vi "Ethernet TCP Engine.vi"(8 "error in (no error)":errorcluster, 9 "Mode":u8, 10 "Engine Name":string, 11 "Varient Data":variant) -> (0 "error out":errorcluster)   [LabVIEW 2024]
doc: "All Rights Reserved © 2023 SyncSols"
uses:
  Main Engine/Controls/Main Engine Engine No.Options.ctl
  TCP Engine/Controls/TCP Engine Serial Interupt Cluster.ctl
  TCP Engine/TCP Engine.lvlib
  Main Engine/Controls/Main Engine Config Confirmation Cluster.ctl
  Controls/Ethernet Dynamic Data Cluster.ctl
  Controls/Ethernet Message Info Cluster.ctl
  Controls/Ethernet Frame Info Cluster.ctl
  Controls/Ethernet Configuration Cluster.ctl
  Controls/Ethernet Command Q Cluster.ctl
  Controls/Ethernet TCP Read Write References.ctl
  Controls/Ethernet State Machine Cases.ctl
  Controls/Ethernet Client Info Cluster.ctl
  Controls/Ethernet Server Listen Loop Cluster.ctl
  Controls/Ethernet Client Info Q Cluster.ctl
  Main Engine/Controls/Main Engine Q Option.ctl
  Main Engine/Controls/Main Engine JSON Command State.ctl
  Controls/Ethernet TCP State Machine Data Cluster.ctl
panel:
  in  "Data Cluster":T1={"Varient Data"=variant(string ""), "Stop Notification"=refnum, "Start Notification"=refnum, "Main Engine Response Q"=refnum, "TCP Engine Response Q"=refnum, "Engine Name"="", "Log File Refnum"=refnum, "Interupt Q"=refnum, "Mode"=0, "Ethernet Configuration"={"Mode"=255, "Local IP"="", "Local Port"=8, "Frame Info"=[], "Minor Frame Freq"=0}, "UDP Connection ID"=refnum, "Command Q"=refnum, "TCP Connection ID"=refnum, "Listener ID"=refnum, "Wait for Listner"=FALSE, "Remote address"=[], "Remote port"=[], "Connection ID"=[], "Client IP"="", "Client Port"=0, "Client Info Q"=refnum, "Server Listen Loop Q"=refnum}
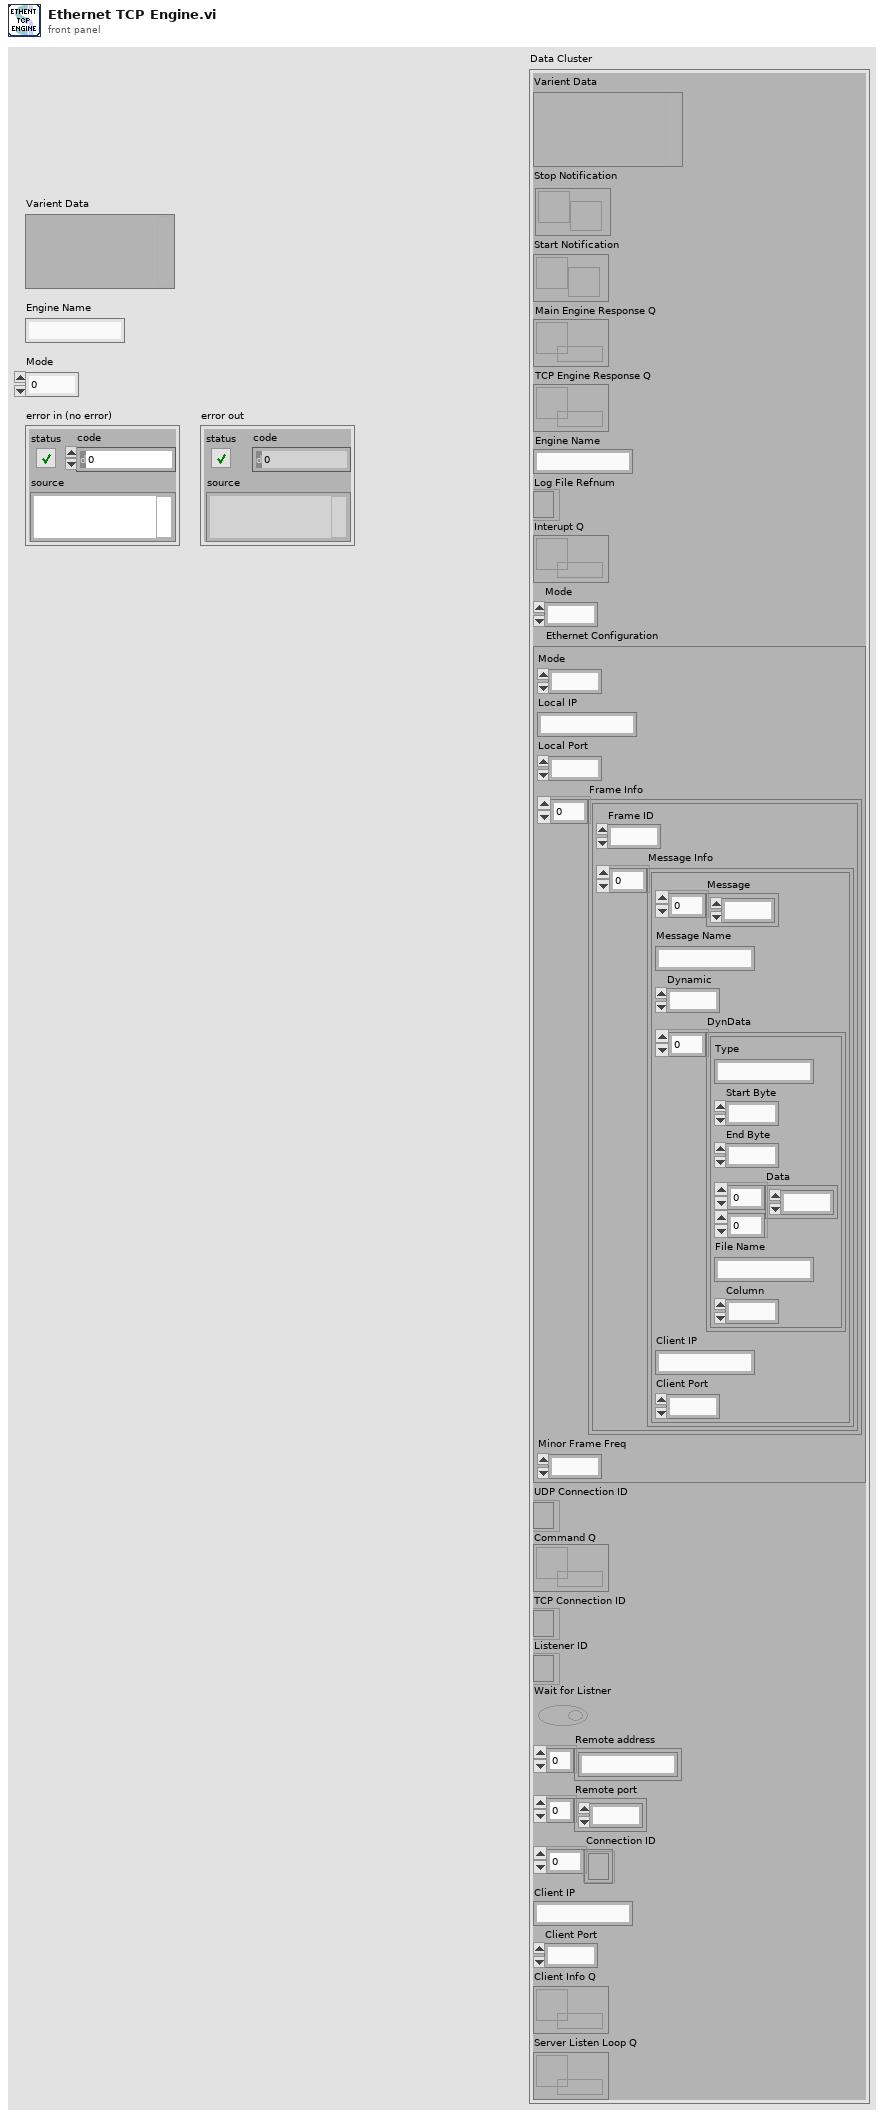
[diagram p1: front panel]
types:
  T1 = typedef "Ethernet TCP State Machine Data Cluster.ctl" = cluster{"Varient Data":variant, "Stop Notification":refnum<notifier>, "Start Notification":refnum<notifier>, "Main Engine Response Q":refnum<queue>, "TCP Engine Response Q":refnum<queue>, "Engine Name":string, "Log File Refnum":refnum<file>, "Interupt Q":refnum<queue>, "Mode":u8, "Ethernet Configuration":T2, "UDP Connection ID":refnum<k16>, "Command Q":refnum<queue>, "TCP Connection ID":refnum<k5>, "Listener ID":refnum<k5>, "Wait for Listner":bool, "Remote address":string[], "Remote port":u16[], "Connection ID":refnum<k5>[], "Client IP":string, "Client Port":u16, "Client Info Q":refnum<queue>, "Server Listen Loop Q":refnum<queue>}
  T2 = typedef "Ethernet Configuration Cluster.ctl" = cluster{"Mode":u8, "Local IP":string, "Local Port":u16, "Frame Info":T3[], "Minor Frame Freq":u8}
  T3 = typedef "Ethernet Frame Info Cluster.ctl" = cluster{"Frame ID":u16, "Message Info":T4[]}
  T4 = typedef "Ethernet Message Info Cluster.ctl" = cluster{"Message":u8[], "Message Name":string, "Dynamic":u8, "DynData":T5[], "Client IP":string, "Client Port":u16}
  T5 = typedef "Ethernet Dynamic Data Cluster.ctl" = cluster{"Type":string, "Start Byte":u8, "End Byte":u8, "Data":u32[][], "File Name":string, "Column":i32}
  T6 = typedef "Ethernet State Machine Cases.ctl" = enum16{">Poll", ".........State Machine.........", ">Init", ">Error", ">Exit", "..........Async Serial..........", ">JSON to LVData", ">Gen Dyn Data", ">Configure", ">Wait for Listener", ">Get Command", ">Write Data"}
  T7 = typedef "Ethernet Server Listen Loop Cluster.ctl" = cluster{"Local IP":string, "References":T8, "Server":bool, "Local Port":u16}
  T8 = typedef "Ethernet TCP Read Write References.ctl" = cluster{"TCP Connection ID":refnum<k5>, "TCP Engine Response Q":refnum<queue>, "Interupt Q":refnum<queue>, "Main Engine Response Q":refnum<queue>, "Stop Notification":refnum<notifier>, "Client Info Q":refnum<queue>}
  T9 = typedef "Main Engine.lvlib/Main Engine Q Option.ctl" = enum16{"Init", "Get"}
  T10 = typedef "Ethernet Client Info Q Cluster.ctl" = cluster{"TCP  ID":refnum<k5>, "Remote port":u16, "Remote IP":string}
  T11 = typedef "TCP Engine.lvlib/TCP Engine Serial Interupt Cluster.ctl" = cluster{"Stop":bool, "JSON Variant":variant}
  T12 = typedef "Ethernet Command Q Cluster.ctl" = cluster{"Ethernet Configuration":T2, "Command State":T13}
  T13 = typedef "Main Engine JSON Command State.ctl" = enum16{"Configure", "Start", "Exit"}
  T14 = typedef "Main Engine.lvlib/Main Engine Engine No.Options.ctl" = enum16{"Init", "Update", "Response", "Get"}
  T15 = typedef "Main Engine.lvlib/Main Engine Config Confirmation Cluster.ctl" = cluster{"Command":string, "Interface":string, "Status":string, "Board":string}
  T16 = typedef "Ethernet Client Info Cluster.ctl" = cluster{"Remote port":u16, "Remote IP":string, "Local port":u16, "Local address":string}
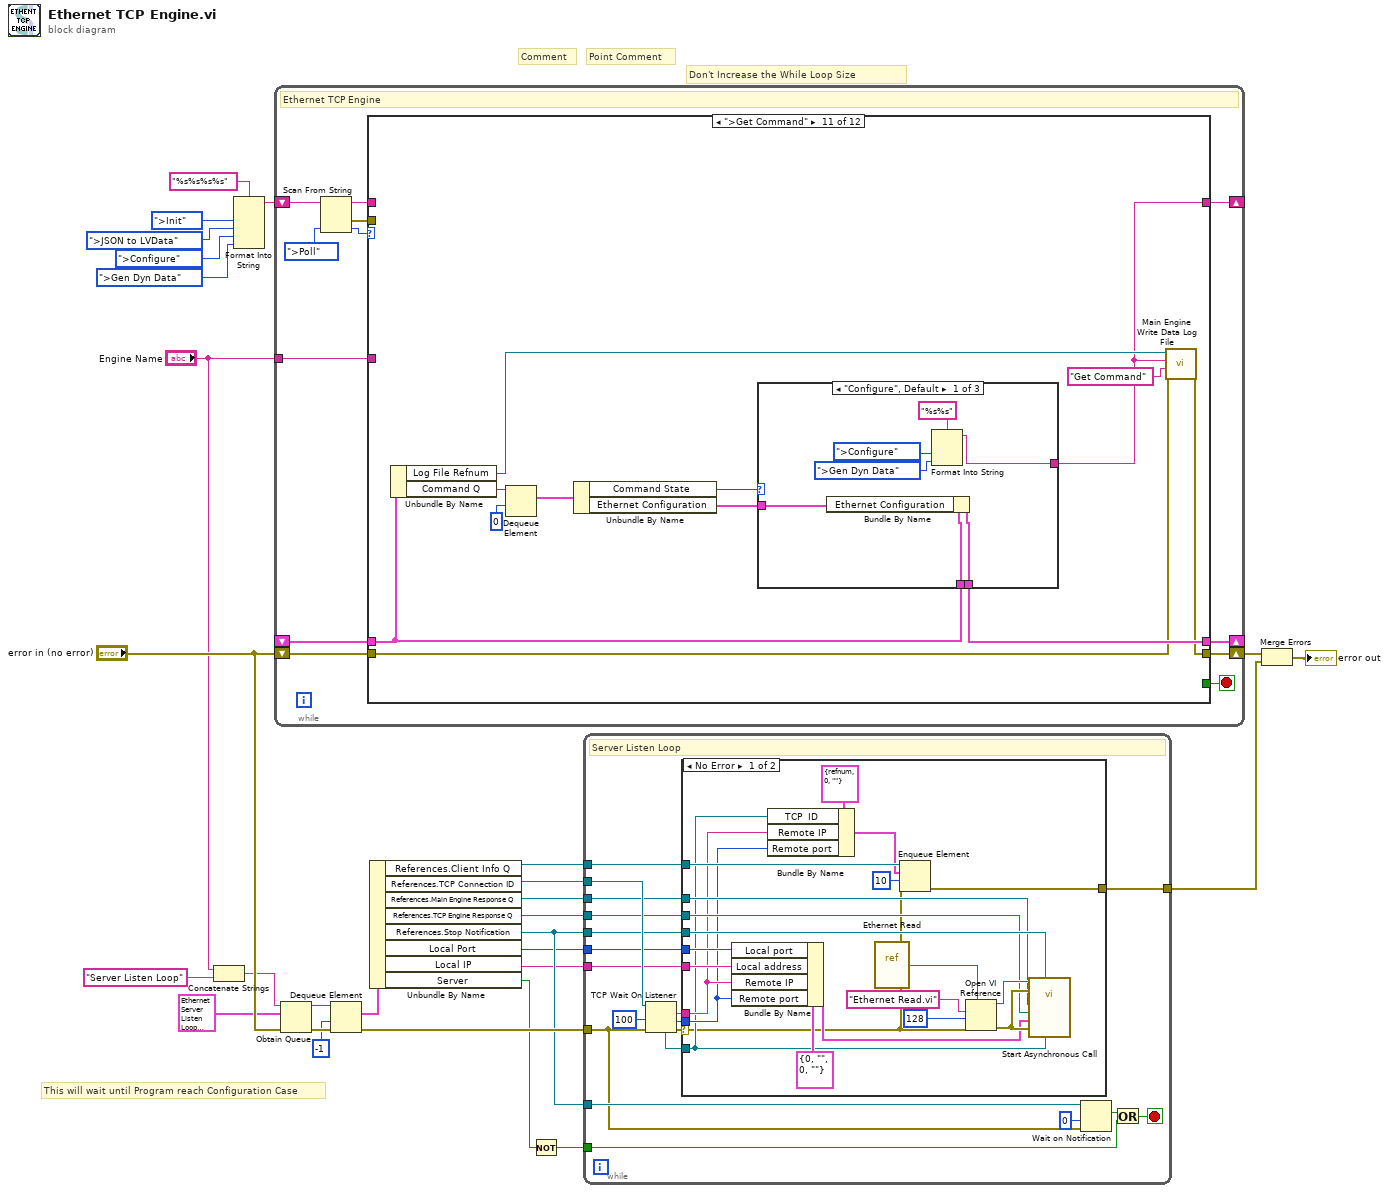
[diagram p0: block diagram]
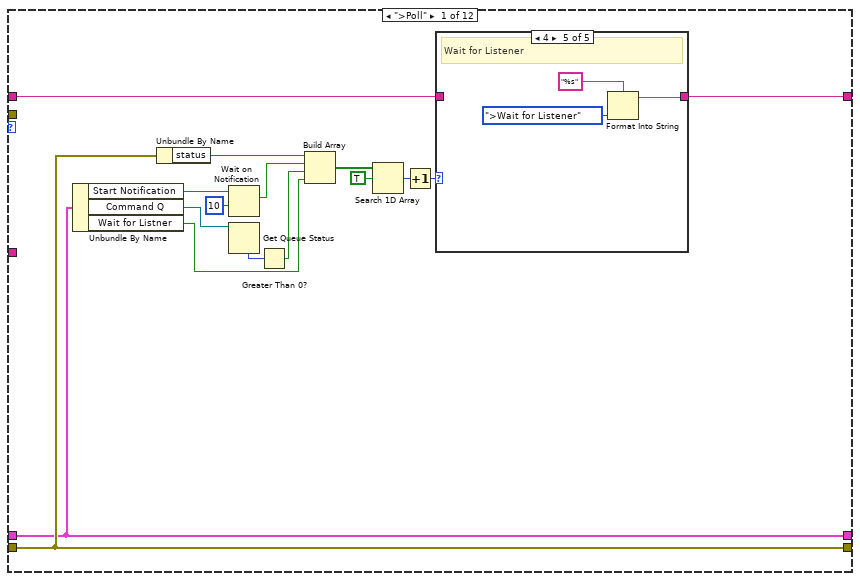
[diagram p3: hidden frame]
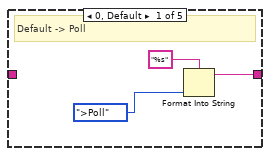
[diagram p4: hidden frame]
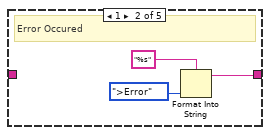
[diagram p5: hidden frame]
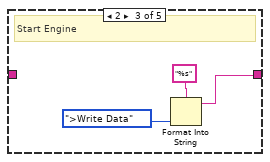
[diagram p6: hidden frame]
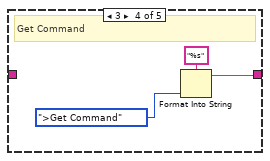
[diagram p7: hidden frame]
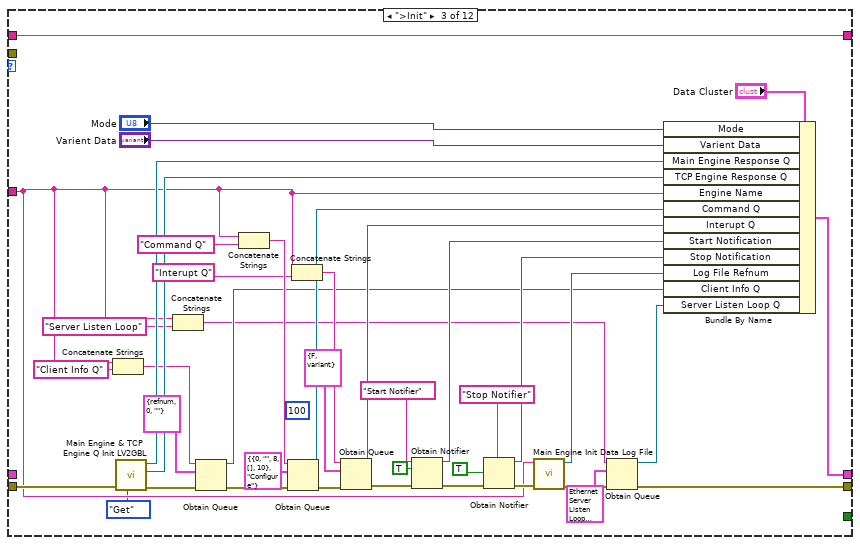
[diagram p9: hidden frame]
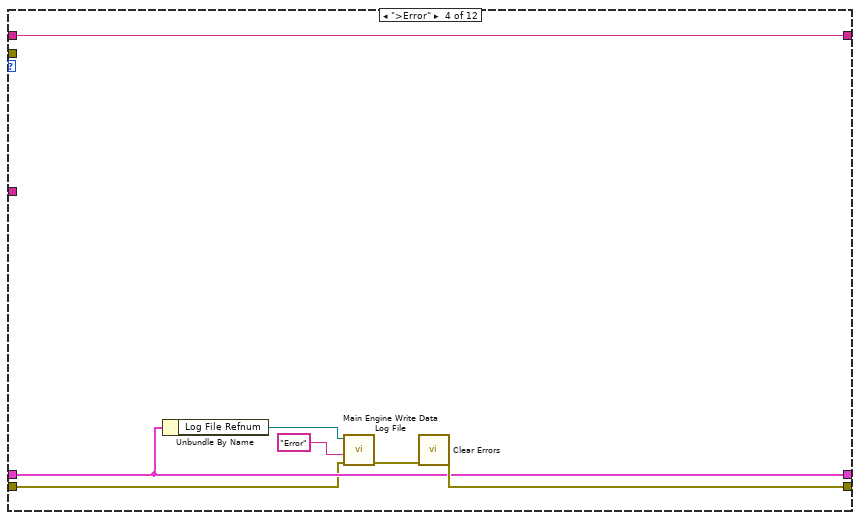
[diagram p10: hidden frame]
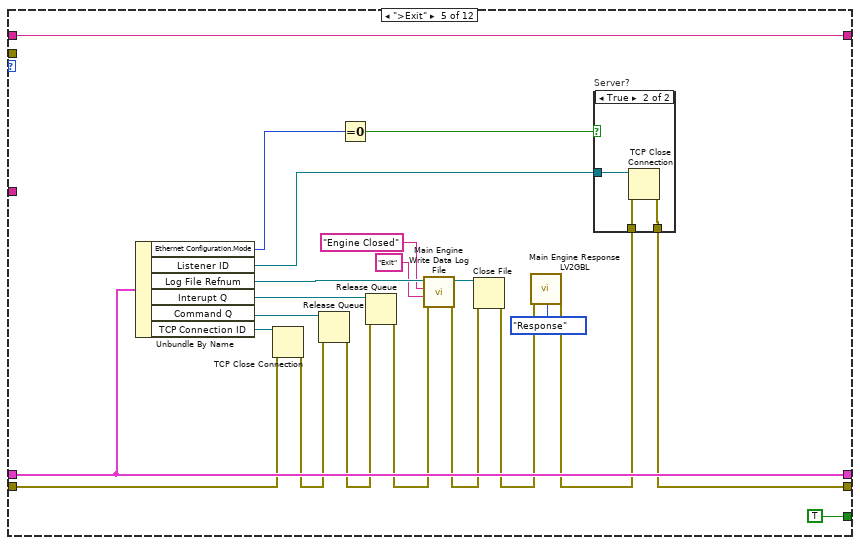
[diagram p11: hidden frame]
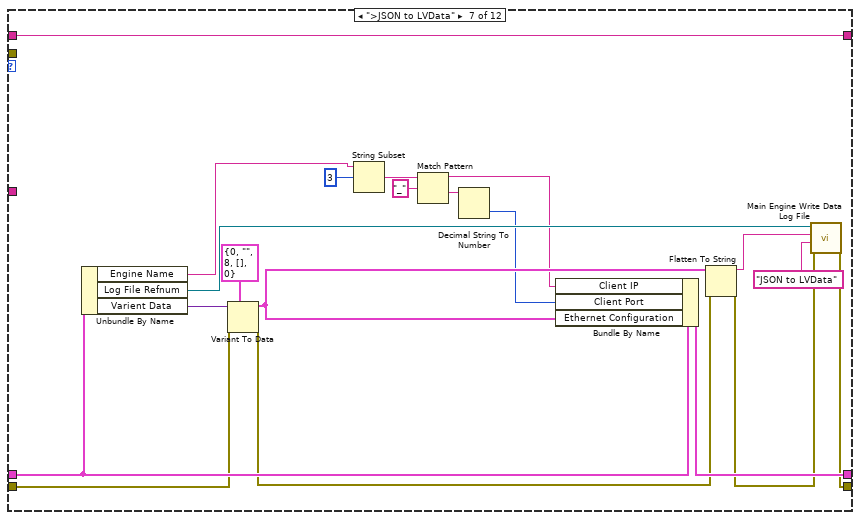
[diagram p14: hidden frame]
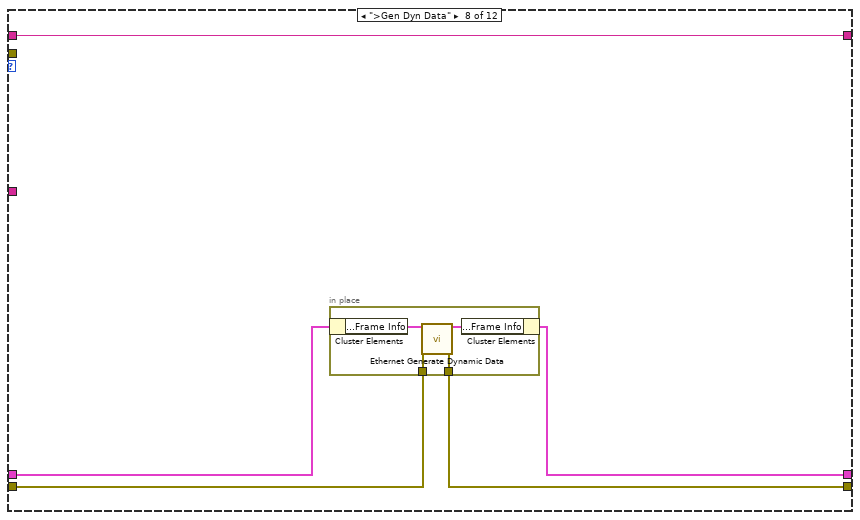
[diagram p15: hidden frame]
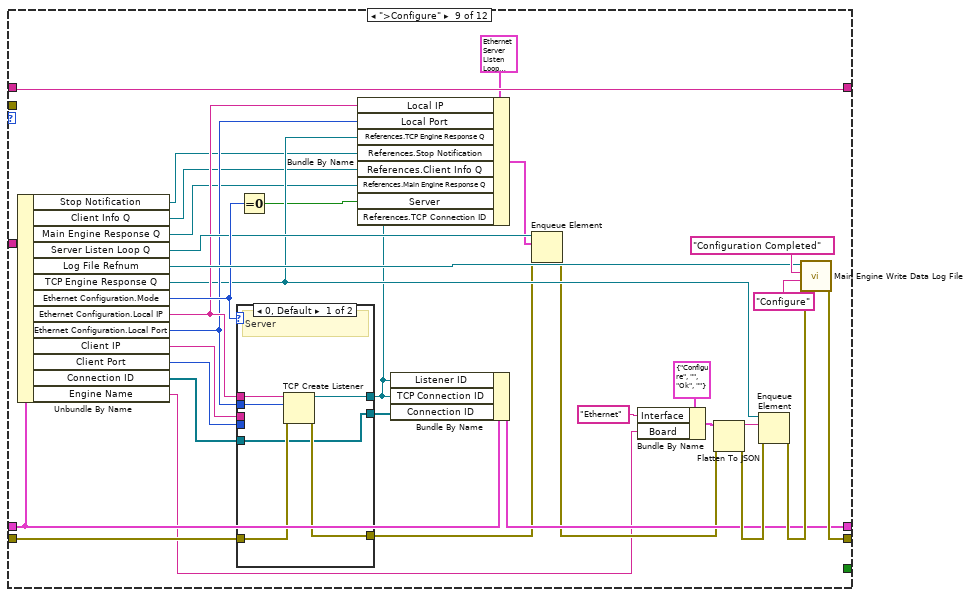
[diagram p16: hidden frame]
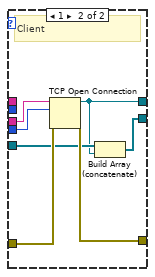
[diagram p17: hidden frame]
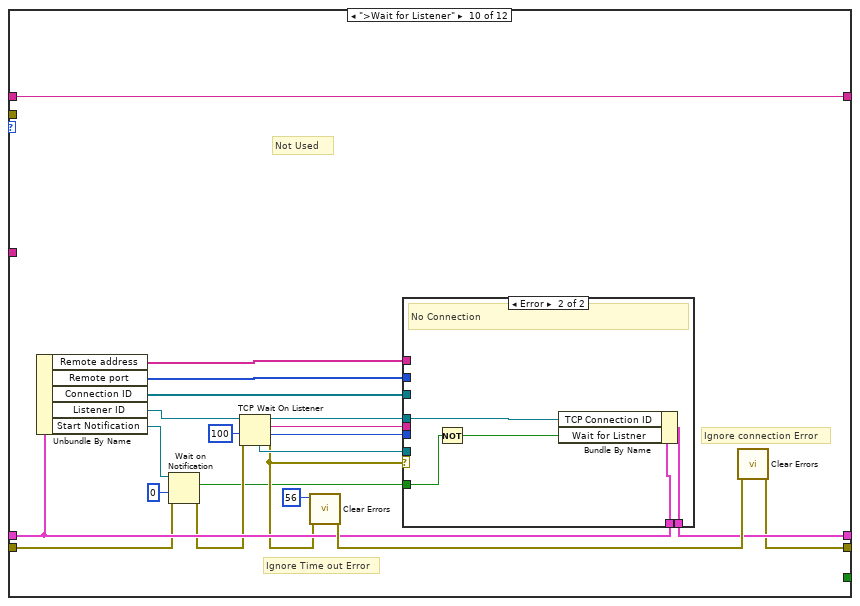
[diagram p18: hidden frame]
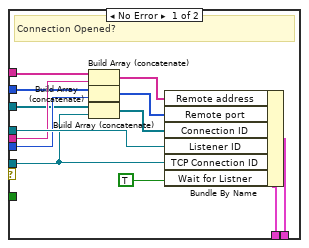
[diagram p19: hidden frame]
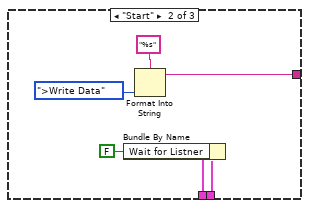
[diagram p20: hidden frame]
diagram:
  # "This will wait until Program reach Configuration Case"
  # "Don't Increase the While Loop Size"
  # "Point Comment"
  # "Comment"
  n1 = Concatenate Strings("Engine Name", "Server Listen Loop" ("string")) -> (w17:string)
  n2 = Format Into String(format string="%s%s%s%s", Ethernet_State_Machine_Cases.">Init" ("SM Cases Options"), Ethernet_State_Machine_Cases.">JSON to LVData" ("SM Cases Options"), Ethernet_State_Machine_Cases.">Configure" ("SM Cases Options"), Ethernet_State_Machine_Cases.">Gen Dyn Data" ("SM Cases Options")) -> (resulting string=w27:string)  [unwired: 2 in, 1 out]
  n3 = while {
    shift-right: [w36] -> _
    shift-left: w27 -> [w40]
    shift-right: [w34] -> w25
    shift-left: "error in (no error)" -> [w35]
    shift-right: [w32] -> _
    shift-left: _ -> [w31]
    tunnel: "Engine Name" -> [w29]
    stop <- w33 stop-if-true
    # "Ethernet TCP Engine"
    n4 = Scan From String(input string=w40, default 1=Ethernet_State_Machine_Cases.">Poll" ("SM Cases Options")) -> (remaining string=w37:string, error out=w39:errorcluster, output 1=w38:T6)  [unwired: 3 in, 1 out]
    n5 = case shown="\">Get Command\"" w38 {
      tunnel: w39 -> [_ _ _ _ _ _ _ _ _ _ _ _]
      tunnel: w37 -> [w56 w74 w115 w122 w144 w151 w171 w176 w195 w247 _ w334]
      tunnel: [w55 w74 w115 w122 w144 w151 w171 w176 w195 w247 w269 w334] -> w36
      tunnel: w35 -> [w54 w73 w93 w117 w134 w150 w161 w174 w202 w235 w266 w327]
      tunnel: [w54 w73 w77 w121 w123 w150 w166 w172 w211 w238 w267 w332] -> w34
      tunnel: [_ _ _ _ TRUE _ _ _ _ _ _ _] -> w33
      tunnel: [w48 w72 w100 w118 w142 w149 w168 w173 w201 w239 w272 w333] -> w32
      tunnel: w31 -> [w48 w72 _ w118 w142 w149 w170 w175 w213 w240 w271 w333]
      tunnel: w29 -> [_ _ w79 _ _ _ _ _ _ _ _ _]
      frame ">Poll" {
        n6 = Unbundle By Name(w48) -> ("Start Notification"=w47:refnum<notifier>, "Command Q"=w46:refnum<queue>, "Wait for Listner"=w41:bool)
        n7 = Unbundle By Name(w54) -> ("status"=w53:bool)
        n8 = Wait on Notification(notifier=w47, timeout in ms (-1)=10) -> (notification=w42:bool)  [unwired: 2 in, 3 out]
        n9 = Get Queue Status(queue=w46) -> (# elements in queue=w44:i32)  [unwired: 2 in, 7 out]
        n10 = Greater Than 0?(x=w44) -> (x > 0?=w43:bool)
        n11 = Build Array(w53, w42, w43, w41) -> (w52:bool[])
        n12 = Search 1D Array(1D array=w52, element=TRUE) -> (index of element=w50:i32)  [unwired: 1 in]
        n13 = Increment(x=w50) -> (x+1=w49:i32)
        n14 = case shown="4" w49 {
          tunnel: w56 -> [_ _ _ _ _]
          tunnel: [w58 w61 w65 w67 w70] -> w55
          frame 0, Default {
            # "Default -> Poll"
            n15 = Format Into String(format string="%s", Ethernet_State_Machine_Cases.">Poll" ("SM Cases Options")) -> (resulting string=w58:string)  [unwired: 2 in, 1 out]
          }
          frame 1 {
            # "Error Occured"
            n16 = Format Into String(format string="%s", Ethernet_State_Machine_Cases.">Error" ("SM Cases Options")) -> (resulting string=w61:string)  [unwired: 2 in, 1 out]
          }
          frame 2 {
            # "Start Engine"
            n17 = Format Into String(format string="%s", Ethernet_State_Machine_Cases.">Write Data" ("SM Cases Options")) -> (resulting string=w65:string)  [unwired: 2 in, 1 out]
          }
          frame 3 {
            # "Get Command"
            n18 = Format Into String(format string="%s", Ethernet_State_Machine_Cases.">Get Command" ("SM Cases Options")) -> (resulting string=w67:string)  [unwired: 2 in, 1 out]
          }
          frame 4 {
            # "Wait for Listener"
            n19 = Format Into String(format string="%s", Ethernet_State_Machine_Cases.">Wait for Listener" ("SM Cases Options")) -> (resulting string=w70:string)  [unwired: 2 in, 1 out]
          }
        }
      }
      frame ".........State Machine........." {
      }
      frame ">Init" {
        (unwired) 100 ("max queue size (-1, unlimited)")
        n20 = Concatenate Strings(w79, "Client Info Q" ("string")) -> (w84:string)
        n21 = call "Main Engine & TCP Engine Q Init LV2GBL.vi"("Q Option"=Main_Engine_Q_Option."Get", "error in"=w93) -> ("error out"=w88:errorcluster, "TCP Enigine Q"=w91:refnum<queue>, "Main Engine Q"=w92:refnum<queue>)  [unwired: 7 in]
        n22 = Concatenate Strings(w79, "Server Listen Loop" ("string")) -> (w82:string)
        n23 = Obtain Queue(name (unnamed)=w84, element data type=T10 {"TCP  ID"=refnum, "Remote port"=0, "Remote IP"=""} ("Client Info Q Cluster"), error in (no error)=w88) -> (queue out=w83:refnum<queue>, error out=w87:errorcluster)  [unwired: 2 in, 1 out]
        n24 = Concatenate Strings(w79, "Command Q" ("name (unnamed)")) -> (w105:string)
        n25 = Obtain Queue(name (unnamed)=w105, element data type=T12 {"Ethernet Configuration"={"Mode"=0, "Local IP"="", "Local Port"=8, "Frame Info"=[], "Minor Frame Freq"=10}, "Command State"=enum."Configure"} ("Async Serial Command Q Cluster"), error in (no error)=w87) -> (queue out=w89:refnum<queue>, error out=w113:errorcluster)  [unwired: 2 in, 1 out]
        n26 = Concatenate Strings(w79, "Interupt Q" ("name (unnamed)")) -> (w103:string)
        n27 = Obtain Queue(name (unnamed)=w103, element data type=T11 {"Stop"=FALSE, "JSON Variant"=variant} ("Serial Interupt Cluster"), error in (no error)=w113) -> (queue out=w94:refnum<queue>, error out=w112:errorcluster)  [unwired: 2 in, 1 out]
        n28 = Obtain Notifier(name (unnamed)="Start Notifier", notification data type=TRUE, error in (no error)=w112) -> (notifier out=w98:refnum<notifier>, error out=w111:errorcluster)  [unwired: 1 in, 1 out]
        n29 = Obtain Notifier(name (unnamed)="Stop Notifier", notification data type=TRUE, error in (no error)=w111) -> (notifier out=w97:refnum<notifier>, error out=w102:errorcluster)  [unwired: 1 in, 1 out]
        n30 = call "Main Engine Init Data Log File.vi"("error in"=w102, "Engine Name"=w79) -> ("error out"=w78:errorcluster, "File Refnum"=w96:refnum<file>)  [unwired: 8 in]
        n31 = Obtain Queue(name (unnamed)=w82, element data type=T7 {"Local IP"="", "References"={"TCP Connection ID"=refnum, "TCP Engine Response Q"=refnum, "Interupt Q"=refnum, "Main Engine Response Q"=refnum, "Stop Notification"=refnum, "Client Info Q"=refnum}, "Server"=FALSE, "Local Port"=0} ("Server Listen Loop Cluster"), error in (no error)=w78) -> (queue out=w76:refnum<queue>, error out=w77:errorcluster)  [unwired: 2 in, 1 out]
        n32 = Bundle By Name(cluster="Data Cluster", "Mode"="Mode", "Varient Data"="Varient Data", "Main Engine Response Q"=w92, "TCP Engine Response Q"=w91, "Engine Name"=w79, "Command Q"=w89, "Interupt Q"=w94, "Start Notification"=w98, "Stop Notification"=w97, "Log File Refnum"=w96, "Client Info Q"=w83, "Server Listen Loop Q"=w76) -> (w100:T1)
      }
      frame ">Error" {
        n33 = Unbundle By Name(w118) -> ("Log File Refnum"=w120:refnum<file>)
        n34 = call "Main Engine Write Data Log File.vi"("error in"=w117, "State"="Error" ("Input Data"), "File Refnum"=w120) -> ("error out"=w116:errorcluster)  [unwired: 7 in, 1 out]
        n35 = call <vilib>:"Clear Errors.vi"("error in (no error)"=w116) -> ("error out"=w121:errorcluster)  [unwired: 5 in, 1 out]
      }
      frame ">Exit" {
        n36 = Unbundle By Name(w142) -> ("Ethernet Configuration.Mode"=w127:u8, "Listener ID"=w125:refnum<k5>, "Log File Refnum"=w138:refnum<file>, "Interupt Q"=w129:refnum<queue>, "Command Q"=w139:refnum<queue>, "TCP Connection ID"=w128:refnum<k5>)
        n37 = TCP Close Connection(connection ID=w128, error in (no error)=w134) -> (error out=w141:errorcluster)  [unwired: 1 in, 1 out]
        n38 = Release Queue(queue=w139, error in (no error)=w141) -> (error out=w140:errorcluster)  [unwired: 1 in, 2 out]
        n39 = Equal To 0?(x=w127) -> (x = 0?=w126:bool)
        n40 = Release Queue(queue=w129, error in (no error)=w140) -> (error out=w137:errorcluster)  [unwired: 1 in, 2 out]
        n41 = call "Main Engine Write Data Log File.vi"("error in"=w137, "State"="Exit", "Input Data"="Engine Closed", "File Refnum"=w138) -> ("error out"=w136:errorcluster, "File Refnum"=w135:refnum<file>)  [unwired: 6 in]
        n42 = Close File(refnum=w135, error in=w136) -> (error out=w131:errorcluster)  [unwired: 1 out]
        n43 = call "Main Engine Response LV2GBL.vi"("Options"=Main_Engine_Engine_No.Options."Response", "error in"=w131) -> ("error out"=w124:errorcluster)  [unwired: 7 in, 2 out]
        n44 = case "Server?" shown="True" w126 {
          tunnel: w125 -> [_ w148]
          tunnel: w124 -> [w145 w147]
          tunnel: [w145 w146] -> w123
          frame False {
          }
          frame True {
            n45 = TCP Close Connection(connection ID=w148, error in (no error)=w147) -> (error out=w146:errorcluster)  [unwired: 1 in, 1 out]
          }
        }
      }
      frame "..........Async Serial.........." {
      }
      frame ">JSON to LVData" {
        n46 = Unbundle By Name(w170) -> ("Engine Name"=w155:string, "Log File Refnum"=w167:refnum<file>, "Varient Data"=w169:variant)
        n47 = Variant To Data(error in=w161, type=T2 {"Mode"=0, "Local IP"="", "Local Port"=8, "Frame Info"=[], "Minor Frame Freq"=0} ("Ethernet Configuration"), Variant=w169) -> (data=w159:T2, error out=w160:errorcluster)
        n48 = String Subset(string=w155, offset (0)=3) -> (substring=w157:string)  [unwired: 1 in]
        n49 = Match Pattern(string=w157, regular expression="_") -> (before substring=w153:string, after substring=w154:string)  [unwired: 1 in, 2 out]
        n50 = Decimal String To Number(string=w154) -> (number=w152:i32)  [unwired: 2 in, 1 out]
        n51 = Bundle By Name(cluster=w170, "Client IP"=w153, "Client Port"=w152, "Ethernet Configuration"=w159) -> (w168:T1)
        n52 = Flatten To String(anything=w159, error in (no error)=w160) -> (data string=w163:string, error out=w164:errorcluster)  [unwired: 2 in, 1 out]
        n53 = call "Main Engine Write Data Log File.vi"("error in"=w164, "State"="JSON to LVData", "Input Data"=w163, "File Refnum"=w167) -> ("error out"=w166:errorcluster)  [unwired: 6 in, 1 out]
      }
      frame ">Gen Dyn Data" {
        n54 = in-place {
          in-place-border: w174 -> [w180]
          in-place-border: [w179] -> w172
          n55 = in-place-cluster #1(w175) -> ("Ethernet Configuration.Frame Info"=w178:T3[])
          n56 = call "Ethernet Generate Dynamic Data.vi"("error in"=w180, "Frame Info"=w178) -> ("error out"=w179:errorcluster, "Frame Info"=w177:T3[])  [unwired: 8 in]
          n57 = in-place-cluster #1("Ethernet Configuration.Frame Info"=w177) -> (w173:T1)
        }
      }
      frame ">Configure" {
        n58 = Unbundle By Name(w213) -> ("Stop Notification"=w186:refnum<notifier>, "Client Info Q"=w188:refnum<queue>, "Main Engine Response Q"=w187:refnum<queue>, "Server Listen Loop Q"=w194:refnum<queue>, "Log File Refnum"=w203:refnum<file>, "TCP Engine Response Q"=w190:refnum<queue>, "Ethernet Configuration.Mode"=w200:u8, "Ethernet Configuration.Local IP"=w192:string, "Ethernet Configuration.Local Port"=w191:u16, "Client IP"=w199:string, "Client Port"=w198:u16, "Connection ID"=w197:refnum<k5>[], "Engine Name"=w181:string)
        n59 = case shown="0, Default" w200 {
          tunnel: w202 -> [w219 w226]
          tunnel: w192 -> [w218 _]
          tunnel: w191 -> [w217 _]
          tunnel: [w216 w225] -> w183
          tunnel: [w215 w223] -> w184
          tunnel: w199 -> [_ w221]
          tunnel: w198 -> [_ w220]
          tunnel: w197 -> [w214 w224]
          tunnel: [w214 w222] -> w196
          frame 0, Default {
            # "Server"
            n60 = TCP Create Listener(8:w219, 10:w217, 11:w218) -> (0:w216:errorcluster, 3:w215:refnum<k5>)  [unwired: 2 in, 1 out]
          }
          frame 1 {
            # "Client"
            n61 = TCP Open Connection(address=w221, remote port or service name=w220, error in (no error)=w226) -> (connection ID=w223:refnum<k5>, error out=w225:errorcluster)  [unwired: 2 in]
            n62 = Build Array (concatenate)(w224, w223) -> (w222:refnum<k5>[])
          }
        }
        n63 = Equal To 0?(x=w200) -> (x = 0?=w185:bool)
        n64 = Bundle By Name(cluster=T7 {"Local IP"="", "References"={"TCP Connection ID"=refnum, "TCP Engine Response Q"=refnum, "Interupt Q"=refnum, "Main Engine Response Q"=refnum, "Stop Notification"=refnum, "Client Info Q"=refnum}, "Server"=FALSE, "Local Port"=0} ("element"), "Local IP"=w192, "Local Port"=w191, "References.TCP Engine Response Q"=w190, "References.Stop Notification"=w186, "References.Client Info Q"=w188, "References.Main Engine Response Q"=w187, "Server"=w185, "References.TCP Connection ID"=w184) -> (w189:T7)
        n65 = Bundle By Name(cluster=w213, "Listener ID"=w184, "TCP Connection ID"=w184, "Connection ID"=w196) -> (w201:T1)
        n66 = Enqueue Element(queue=w194, element=w189, error in (no error)=w183) -> (error out=w182:errorcluster)  [unwired: 1 in, 2 out]
        n67 = Bundle By Name(cluster=T15 {"Command"="Configure", "Interface"="", "Status"="Ok", "Board"=""}, "Interface"="Ethernet" ("SubCmd"), "Board"=w181) -> (w209:T15)
        n68 = Flatten To JSON(anything=w209, error in (no error)=w182) -> (JSON string=w208:string, 11:w205:errorcluster)  [unwired: 1 in]
        n69 = Enqueue Element(queue=w190, element=w208, error in (no error)=w205) -> (error out=w204:errorcluster)  [unwired: 1 in, 2 out]
        n70 = call "Main Engine Write Data Log File.vi"("error in"=w204, "State"="Configure", "Input Data"="Configuration Completed", "File Refnum"=w203) -> ("error out"=w211:errorcluster)  [unwired: 6 in, 1 out]
      }
      frame ">Wait for Listener" {
        # "Not Used"
        # "Ignore connection Error"
        # "Ignore Time out Error"
        n71 = Unbundle By Name(w240) -> ("Remote address"=w229:string[], "Remote port"=w228:u16[], "Connection ID"=w227:refnum<k5>[], "Listener ID"=w246:refnum<k5>, "Start Notification"=w236:refnum<notifier>)
        n72 = Wait on Notification(notifier=w236, timeout in ms (-1)=0, error in (no error)=w235) -> (notification=w233:bool, error out=w234:errorcluster)  [unwired: 1 in, 2 out]
        n73 = TCP Wait On Listener(8:w234, 9:100 ("timeout ms (wait forever: -1)"), 11:w246) -> (0:w237:errorcluster, 1:w230:u16, 2:w231:string, 3:w242:refnum<k5>, 4:w241:refnum<k5>)  [unwired: 1 in]
        n74 = call <vilib>:"Clear Errors.vi"("error in (no error)"=w237, "specific error code to clear (0: all)"=56) -> ("error out"=w243:errorcluster)  [unwired: 4 in, 1 out]
        n75 = case "Connection Opened?" shown="Error" w237 {
          tunnel: w242 -> [w257 w264]
          tunnel: w241 -> [w251 _]
          tunnel: w240 -> [w259 w265]
          tunnel: [w258 w263] -> w239
          tunnel: w233 -> [_ w262]
          tunnel: w231 -> [w255 _]
          tunnel: w230 -> [w253 _]
          tunnel: w229 -> [w256 _]
          tunnel: w228 -> [w254 _]
          tunnel: w227 -> [w252 _]
          frame No Error {
            # "Connection Opened?"
            n76 = Build Array (concatenate)(w256, w255) -> (w250:string[])
            n77 = Build Array (concatenate)(w254, w253) -> (w249:u16[])
            n78 = Build Array (concatenate)(w252, w251) -> (w248:refnum<k5>[])
            n79 = Bundle By Name(cluster=w259, "Remote address"=w250, "Remote port"=w249, "Connection ID"=w248, "Listener ID"=w257, "TCP Connection ID"=w251, "Wait for Listner"=TRUE ("Wait for Listener?")) -> (w258:T1)
          }
          frame Error {
            # "No Connection"
            n80 = Not(x=w262) -> (.not. x?=w261:bool)
            n81 = Bundle By Name(cluster=w265, "TCP Connection ID"=w264, "Wait for Listner"=w261) -> (w263:T1)
          }
        }
        n82 = call <vilib>:"Clear Errors.vi"("error in (no error)"=w243) -> ("error out"=w238:errorcluster)  [unwired: 5 in, 1 out]
      }
      frame ">Get Command" {
        n83 = Unbundle By Name(w271) -> ("Log File Refnum"=w270:refnum<file>, "Command Q"=w277:refnum<queue>)
        n84 = Dequeue Element(queue=w277, timeout in ms (-1)=0) -> (element=w275:T12)  [unwired: 1 in, 3 out]
        n85 = Unbundle By Name(w275) -> ("Command State"=w274:T13, "Ethernet Configuration"=w273:T2)
        n86 = case shown="\"Configure\", Default" w274 {
          tunnel: w271 -> [w284 w287 w294]
          tunnel: w273 -> [w280 _ _]
          tunnel: [w283 w286 w294] -> w272
          tunnel: [w281 w290 w292] -> w269
          frame "Configure", Default {
            n87 = Bundle By Name(cluster=w284, "Ethernet Configuration"=w280) -> (w283:T1)
            n88 = Format Into String(format string="%s%s", Ethernet_State_Machine_Cases.">Configure" ("SM Cases Options"), Ethernet_State_Machine_Cases.">Gen Dyn Data" ("SM Cases Options")) -> (resulting string=w281:string)  [unwired: 2 in, 1 out]
          }
          frame "Start" {
            n89 = Bundle By Name(cluster=w287, "Wait for Listner"=FALSE) -> (w286:T1)
            n90 = Format Into String(format string="%s", Ethernet_State_Machine_Cases.">Write Data" ("SM Cases Options")) -> (resulting string=w290:string)  [unwired: 2 in, 1 out]
          }
          frame "Exit" {
            n91 = Format Into String(format string="%s", Ethernet_State_Machine_Cases.">Exit" ("SM Cases Options")) -> (resulting string=w292:string)  [unwired: 2 in, 1 out]
          }
        }
        n92 = call "Main Engine Write Data Log File.vi"("error in"=w266, "State"="Get Command", "Input Data"=w269, "File Refnum"=w270) -> ("error out"=w267:errorcluster)  [unwired: 6 in, 1 out]
      }
      frame ">Write Data" {
        n93 = Unbundle By Name(w333) -> ("Ethernet Configuration.Mode"=w298:u8, "Ethernet Configuration.Local Port"=w297:u16, "Ethernet Configuration.Local IP"=w296:string, "Client IP"=w302:string, "Client Port"=w301:u16, "Remote port"=w308:u16[], "Remote address"=w307:string[], "TCP Connection ID"=w315:refnum<k5>, "TCP Engine Response Q"=w314:refnum<queue>, "Interupt Q"=w313:refnum<queue>, "Client Info Q"=w312:refnum<queue>, "Stop Notification"=w311:refnum<notifier>, "Main Engine Response Q"=w299:refnum<queue>, "Ethernet Configuration.Minor Frame Freq"=w317:u8, "Ethernet Configuration.Frame Info"=w318:T3[], "Connection ID"=w309:refnum<k5>[], "Log File Refnum"=w328:refnum<file>)
        n94 = Bundle By Name(cluster=T8 {"TCP Connection ID"=refnum, "TCP Engine Response Q"=refnum, "Interupt Q"=refnum, "Main Engine Response Q"=refnum, "Stop Notification"=refnum, "Client Info Q"=refnum} ("References"), "TCP Connection ID"=w315, "TCP Engine Response Q"=w314, "Interupt Q"=w313, "Client Info Q"=w312, "Stop Notification"=w311, "Main Engine Response Q"=w299) -> (w310:T8)
        n95 = for {
          tunnel: w307 -> [w342] mode=indexing
          tunnel: w308 -> [w341] mode=indexing
          tunnel: [w340] -> w306 mode=indexing
          tunnel: T16 {"Remote port"=0, "Remote IP"="", "Local port"=0, "Local address"=""} -> [w339]
          n96 = Bundle By Name(cluster=w339, "Remote port"=w341, "Remote IP"=w342) -> (w340:T16)
        }
        n97 = call "Main Engine Write Data Log File.vi"("error in"=w327, "State"="Write Data", "Input Data"="Data Read&Write are started", "File Refnum"=w328) -> ("error out"=w319:errorcluster)  [unwired: 6 in, 1 out]
        n98 = Not Equal To 0?(x=w298) -> (x != 0?=w295:bool)
        n99 = Bundle By Name(cluster=T16 {"Remote port"=0, "Remote IP"="", "Local port"=0, "Local address"=""}, "Local port"=w297, "Local address"=w296, "Remote IP"=w302, "Remote port"=w301) -> (w300:T16)
        n100 = case "Client?" shown="True" w295 {
          tunnel: w306 -> [w335 w338]
          tunnel: [w335 w337] -> w305
          tunnel: w300 -> [_ w336]
          frame False {
          }
          frame True {
            n101 = Build Array (concatenate)(w338, w336) -> (w337:T16[])
          }
        }
        n102 = call "Ethernet TCP Read&Write.vi"("Connection ID"=w309, "Client?"=w295, "Frame Info Array"=w318, "Client Info"=w305, "error in"=w319, "Minor Frame Freq"=w317, "References"=w310) -> ("error out"=w321:errorcluster, "Device Stop"=w320:bool)  [unwired: 3 in]
        n103 = Select(t="Device Stop" ("Input Data"), s=w320, f="All Stop" ("Input Data")) -> (s? t:f=w324:string)
        n104 = call <vilib>:"Space Constant.vi"() -> ("String"=w322:string)
        n105 = Concatenate Strings(w324, w322) -> (w323:string)
        n106 = call "Main Engine Write Data Log File.vi"("error in"=w321, "State"="Write Data", "Input Data"=w323, "File Refnum"=w328) -> ("error out"=w332:errorcluster)  [unwired: 6 in, 1 out]
      }
    }
  }
  n107 = Obtain Queue(name (unnamed)=w17, element data type=T7 {"Local IP"="", "References"={"TCP Connection ID"=refnum, "TCP Engine Response Q"=refnum, "Interupt Q"=refnum, "Main Engine Response Q"=refnum, "Stop Notification"=refnum, "Client Info Q"=refnum}, "Server"=FALSE, "Local Port"=0} ("Server Listen Loop Cluster"), error in (no error)="error in (no error)") -> (queue out=w18:refnum<queue>, error out=w20:errorcluster)  [unwired: 2 in, 1 out]
  n108 = Dequeue Element(queue=w18, timeout in ms (-1)=-1, error in (no error)=w20) -> (element=w13:T7, error out=w19:errorcluster)  [unwired: 2 out]
  n109 = Unbundle By Name(w13) -> ("References.Client Info Q"=w4:refnum<queue>, "References.TCP Connection ID"=w12:refnum<k5>, "References.Main Engine Response Q"=w10:refnum<queue>, "References.TCP Engine Response Q"=w9:refnum<queue>, "References.Stop Notification"=w11:refnum<notifier>, "Local Port"=w8:u16, "Local IP"=w7:string, "Server"=w6:bool)
  n110 = Not(x=w6) -> (.not. x?=w5:bool)
  n111 = while {
    tunnel: w19 -> [w352]
    tunnel: w12 -> [w356]
    tunnel: w11 -> [w355]
    tunnel: w11 -> [w351]
    tunnel: w10 -> [w350]
    tunnel: w9 -> [w349]
    tunnel: w8 -> [w348]
    tunnel: w7 -> [w347]
    tunnel: w5 -> [w345]
    tunnel: w4 -> [w344]
    tunnel: [w343] -> w2
    stop <- w346 stop-if-true
    # "Server Listen Loop"
    n112 = TCP Wait On Listener(8:w352, 9:100 ("timeout ms (wait forever: -1)"), 11:w356) -> (0:w360:errorcluster, 1:w358:u16, 2:w359:string, 4:w357:refnum<k5>)  [unwired: 1 in, 1 out]
    n113 = case shown="No Error" w360 {
      selector: w360 -> [w362 _]
      tunnel: w359 -> [w368 _]
      tunnel: w358 -> [w367 _]
      tunnel: w357 -> [w366 _]
      tunnel: w351 -> [w377 _]
      tunnel: w350 -> [w376 _]
      tunnel: w349 -> [w375 _]
      tunnel: w348 -> [w372 _]
      tunnel: w347 -> [w371 _]
      tunnel: w344 -> [w370 _]
      tunnel: [w363 _] -> w343
      frame No Error {
        n114 = Bundle By Name(cluster=T16 {"Remote port"=0, "Remote IP"="", "Local port"=0, "Local address"=""} ("Client Info"), "Local port"=w372, "Local address"=w371, "Remote IP"=w368, "Remote port"=w367) -> (w373:T16)
        n115 = Bundle By Name(cluster=T10 {"TCP  ID"=refnum, "Remote port"=0, "Remote IP"=""} ("element"), "TCP  ID"=w366, "Remote IP"=w368, "Remote port"=w367) -> (w365:T10)
        n116 = vi-ref "Ethernet Read.vi"() -> (w381:refnum<vi>)
        n117 = Enqueue Element(queue=w370, element=w365, timeout in ms (-1)=10, error in (no error)=w362) -> (error out=w363:errorcluster)  [unwired: 2 out]
        n118 = Open VI Reference(type specifier VI Refnum (for type only)=w381, vi path="Ethernet Read.vi", options=128, error in (no error)=w362) -> (vi reference=w382:refnum<vi>, error out=w378:errorcluster)  [unwired: 2 in]
        n119 = call-by-ref "Start Asynchronous Call"(reference=w382, error in=w378, "connection ID"=w366, "Stop Notification"=w377, "error in"=w378, "Client Info"=w373, "TCP Engine Response Q"=w375, "Main Engine Response Q"=w376) -> ()  [unwired: 5 in, 3 out]
      }
      frame Error {
      }
    }
    n120 = Wait on Notification(notifier=w355, timeout in ms (-1)=0, error in (no error)=w352) -> (notification=w354:bool)  [unwired: 1 in, 3 out]
    n121 = Or(x=w354, y=w345) -> (x .or. y?=w346:bool)
  }
  n122 = Merge Errors(w25, w2) -> (→"error out":errorcluster)
